vi "Accelermeter_Final.vi"() -> ()   [LabVIEW 2022 SP3]
uses:
  <vilib>/MakerHub/LINX/Public/Sensors/Accelerometer/MPU60X0/DeviceAddresses.ctl
  <vilib>/MakerHub/LINX/Public/Sensors/Accelerometer/MPU60X0/Clock Source.ctl
  <vilib>/MakerHub/LINX/Public/Utilities/Open Serial.vi
  <vilib>/MakerHub/LINX/Public/Sensors/Accelerometer/MPU60X0/MPU60X0.lvlib
  <vilib>/MakerHub/LINX/LMH-LINX.lvlib
panel:
  out "String":string
  in  "stop":bool
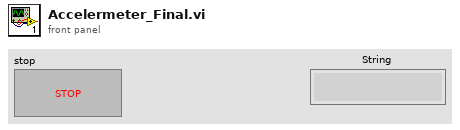
[diagram p1: front panel]
types:
  T1 = typedef "LMH-LINX.lvlib/MPU60X0.lvlib/Clock Source.ctl" = enum8{"Internal 8MHz Osc", "PLL with X Gyro Ref", "PLL with Y Gyro Ref", "PLL with Z Gyro Ref", "PLL with ext 32.768 KHz Ref", "PLL with ext 19.2 MHz Ref", "Reserved", "Hold in reset"}
  T2 = typedef "LMH-LINX.lvlib/MPU60X0.lvlib/DeviceAddresses.ctl" = enum16{"0x68", "0x69"}
  T3 = typedef "LMH-LINX.lvlib/LINX Ref.ctl" = cluster{"IO":T4, "Interface":T5, "LINX Device Config":T6}
  T4 = typedef "LMH-LINX.lvlib/Platform.ctl" = enum16{"Remote", "Local"}
  T5 = typedef "LMH-LINX.lvlib/Interface.ctl" = enum16{"Serial", "TCP"}
  T6 = typedef "LMH-LINX.lvlib/Device.lvlib/LINX Device Config.ctl" = cluster{"Interface":T5, "COM Port":refnum<visa-resource-name>, "TCP Configuration":T7, "Device Family":u8, "Device ID":u8, "Device Name":string, "TCP Ref":refnum<k5>, "Channels":T8}
  T7 = typedef "LMH-LINX.lvlib/Device.lvlib/TCP Config.ctl" = cluster{"IP Address":string, "Port":u16}
  T8 = typedef "LMH-LINX.lvlib/Channels.ctl" = cluster{"DI":u8[], "DO":u8[], "AI":u8[], "AO":u8[], "PWM":u8[], "QE":u8[], "UART":u8[], "I2C 2":u8[], "SPI":u8[], "CAN":u8[], "Servo":u8[], "AI Ref (V)":dbl, "AI Resolution (Bits)":u8, "AO Ref (V)":dbl, "AO Resolution (Bits)":u8}
  T9 = cluster{"X Axis":i16, "Y Axis":i16, "Z Axis":i16}
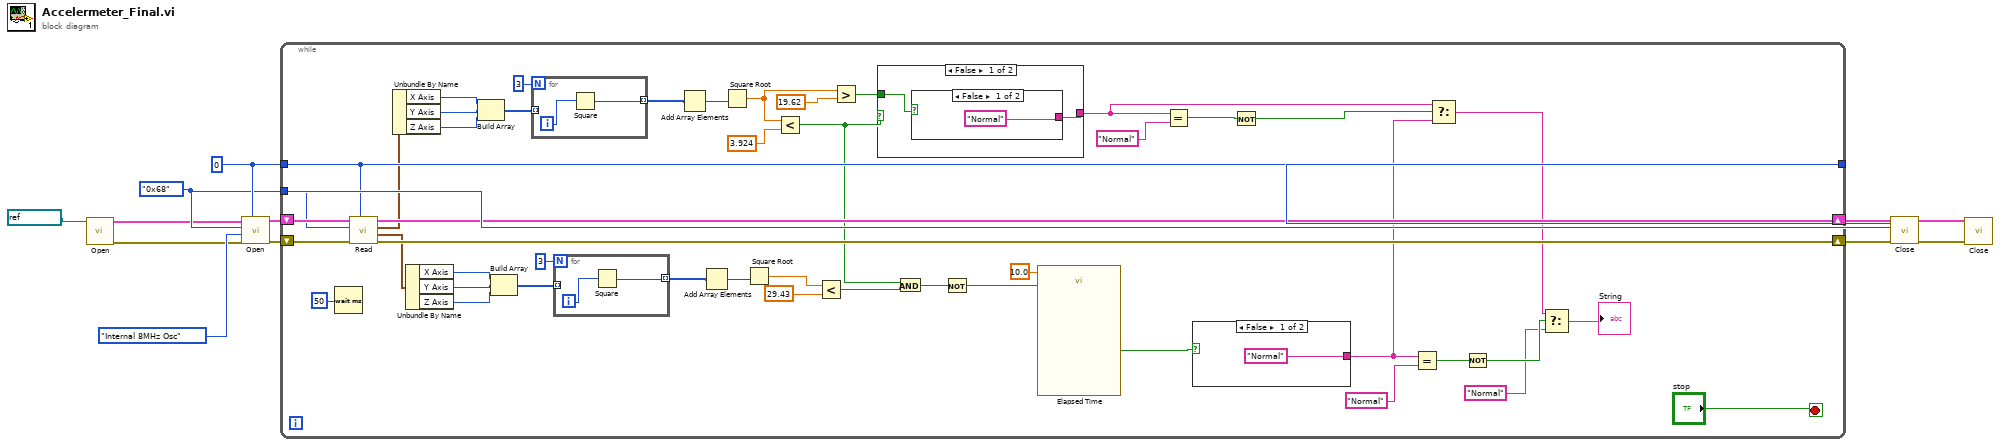
[diagram p0: block diagram]
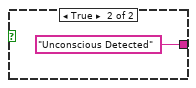
[diagram p2: hidden frame]
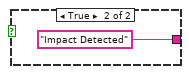
[diagram p3: hidden frame]
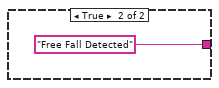
[diagram p4: hidden frame]
diagram:
  w8 = u8 0 ("I2C Channel")
  w7 = DeviceAddresses."0x68" ("I2C Slave Address")
  n1 = call-poly <vilib>:"Open.vi"("Serial Port"=refnum<visa-resource-name> "COM5") -> ("Error Out"=w6:errorcluster, "LINX Resource"=w5:T3)  [unwired: 8 in, 1 out]
  n2 = call <vilib>:"Open.vi"("I2C Channel"=w8, "Error In"=w6, "Clock Source"=Clock_Source."Internal 8MHz Osc", "I2C Slave Address"=w7, "LINX Resource"=w5) -> ("Error Out"=w11:errorcluster, "LINX Resource"=w13:T3)  [unwired: 5 in]
  n3 = while {
    tunnel: w8 -> [w53]
    tunnel: w7 -> [w56]
    shift-right: [w59] -> w12
    shift-left: w13 -> [w60]
    shift-right: [w57] -> w10
    shift-left: w11 -> [w58]
    tunnel: [w53] -> w1
    stop <- "stop" stop-if-true
    n4 = Wait (ms)(milliseconds to wait=u32 50) -> ()  [unwired: 1 out]
    n5 = call <vilib>:"Read.vi"("I2C Channel"=w53, "Error In"=w58, "I2C Slave Address"=w56, "LINX Resource"=w60) -> ("Error Out"=w57:errorcluster, "Gyro  Data (dps)"=w41:T9, "Acceleration Data (g)"=w52:T9, "LINX Resource"=w59:T3)  [unwired: 3 in, 1 out]
    n6 = Unbundle By Name(w52) -> ("X Axis"=w51:i16, "Y Axis"=w50:i16, "Z Axis"=w49:i16)
    n7 = Unbundle By Name(w41) -> ("X Axis"=w44:i16, "Y Axis"=w43:i16, "Z Axis"=w42:i16)
    n8 = Build Array(w51, w50, w49) -> (w47:i16[])
    n9 = Build Array(w44, w43, w42) -> (w37:i16[])
    n10 = for {
      N: 3 -> [_]
      tunnel: w47 -> [_] mode=indexing
      tunnel: [w70] -> w46 mode=indexing
      i -> [w71]
      n11 = Square(x=w71) -> (x^2=w70:i32)
    }
    n12 = for {
      N: 3 -> [_]
      tunnel: [w68] -> w39 mode=indexing
      tunnel: w37 -> [_] mode=indexing
      i -> [w69]
      n13 = Square(x=w69) -> (x^2=w68:i32)
    }
    n14 = Add Array Elements(numeric array=w46) -> (sum=w45:i32)
    n15 = Add Array Elements(numeric array=w39) -> (sum=w38:i32)
    n16 = Square Root(x=w45) -> (sqrt(x)=w35:dbl)
    n17 = Square Root(x=w38) -> (sqrt(x)=w32:dbl)
    n18 = Less?(x=w35, y=3.924) -> (x < y?=w29:bool)
    n19 = Less?(x=w32, y=29.43) -> (x < y?=w30:bool)
    n20 = Greater?(x=w35, y=19.62) -> (0:w33:bool)
    n21 = case shown="False" w29 {
      tunnel: w33 -> [w64 _]
      tunnel: [w63 "Free Fall Detected"] -> w19
      frame False {
        n22 = case shown="False" w64 {
          tunnel: ["Normal" "Impact Detected"] -> w63
          frame False {
          }
          frame True {
          }
        }
      }
      frame True {
      }
    }
    n23 = And(x=w29, y=w30) -> (x .and. y?=w28:bool)
    n24 = Not(x=w28) -> (.not. x?=w27:bool)
    n25 = call "Elapsed Time"("Time Target (s)"=10.0, "Reset"=w27) -> ("Time has Elapsed"=w25:bool)  [unwired: 10 in, 7 out]
    n26 = Equal?(x=w19, y="Normal") -> (x = y?=w22:bool)
    n27 = case shown="False" w25 {
      tunnel: ["Normal" "Unconscious Detected"] -> w18
      frame False {
      }
      frame True {
      }
    }
    n28 = Not(x=w22) -> (.not. x?=w20:bool)
    n29 = Equal?(x=w18, y="Normal") -> (x = y?=w21:bool)
    n30 = Select(t=w19, s=w20, f=w18) -> (s? t:f=w16:string)
    n31 = Not(x=w21) -> (.not. x?=w17:bool)
    n32 = Select(t=w16, s=w17, f="Normal") -> (s? t:f=→"String":string)
  }
  n33 = call <vilib>:"Close.vi"("I2C Channel (0)"=w1, "Error In"=w10, "I2C Slave Address (0)"=w7, "LINX Resource"=w12) -> ("Error Out"=w3:errorcluster, "LINX Resource"=w4:T3)  [unwired: 6 in]
  n34 = call <vilib>:"Close.vi"("Error In"=w3, "LINX Resource"=w4) -> ()  [unwired: 9 in, 1 out]
